vi "Sequence Editor.vi"() -> ()   [LabVIEW 2013, in "Simple Sequence Tools - Editor.lvlib"]
uses:
  Simple Sequence Editor Tool Support.llb/Simple Sequence Tools - Editor.lvlib
  Simple Sequence Editor Tool Support.llb/Simple Sequence Tools - Shared.lvlib
panel:
  in  "Sequence":i32[](listbox)
  in  "NIVS.Workspace Event":refnum<event-registration>
  in  "Iteration Information Channel":string(combo)
  in  "Iterations":u32=1 min=1
  in  "View":enum8{"Step Properties", "Sequence Properties"}(ring)=enum."Sequence Properties"
  in  "Abort Channel":string(combo)
  in  "Step Information Channel":string(combo)
  out "Graph":waveform(dbl)[](graph)
  out "Path":path
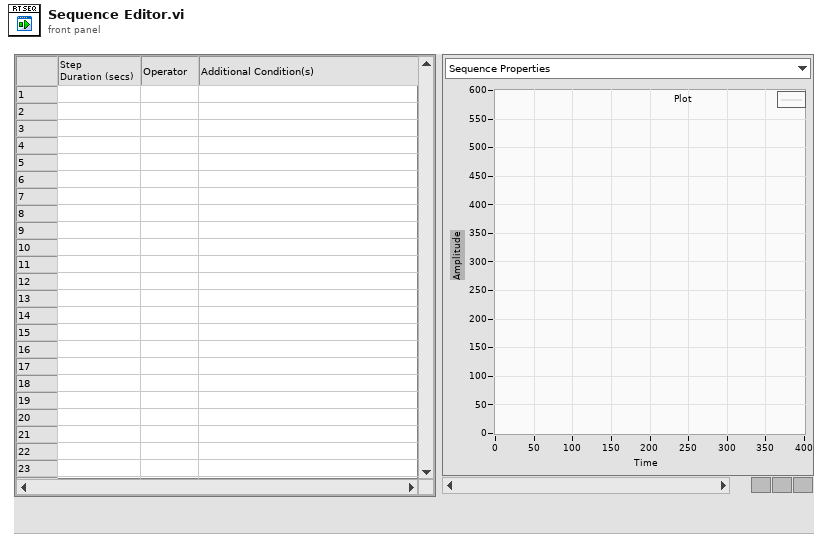
[diagram p1: front panel]
types:
  T1 = cluster{"Aliases.All":cluster{"Name":string, "NodePath":string, "ScaleUnits":string}[], "Aliases.Outputs":cluster{"Name":string, "NodePath":string, "ScaleUnits":string}[], "UI.Sequence#ofColumns":i32, "SysDef.Path":path, "UI.SequenceRef":refnum<vi>, "UI.StepInformationRef":refnum<vi>, "UI.AbortRef":refnum<vi>, "UI.GraphRef":refnum<vi>, "UI.ViewRef":refnum<vi>, "UI.IterationsRef":refnum<vi>, "UI.IterationInformationRef":refnum<vi>, "INI.Settings":cluster{"Build Location":path, "LoggingLocation":path}, "NIVS.Workspace Event":refnum<event-registration>}
  T2 = typedef "LVPoint32TypeDef.ctl" = cluster{"Horizontal":i32, "Vertical":i32}
  T3 = cluster{"Build Location":path, "LoggingLocation":path}
  T4 = cluster{"Name":string, "NodePath":string, "ScaleUnits":string}[]
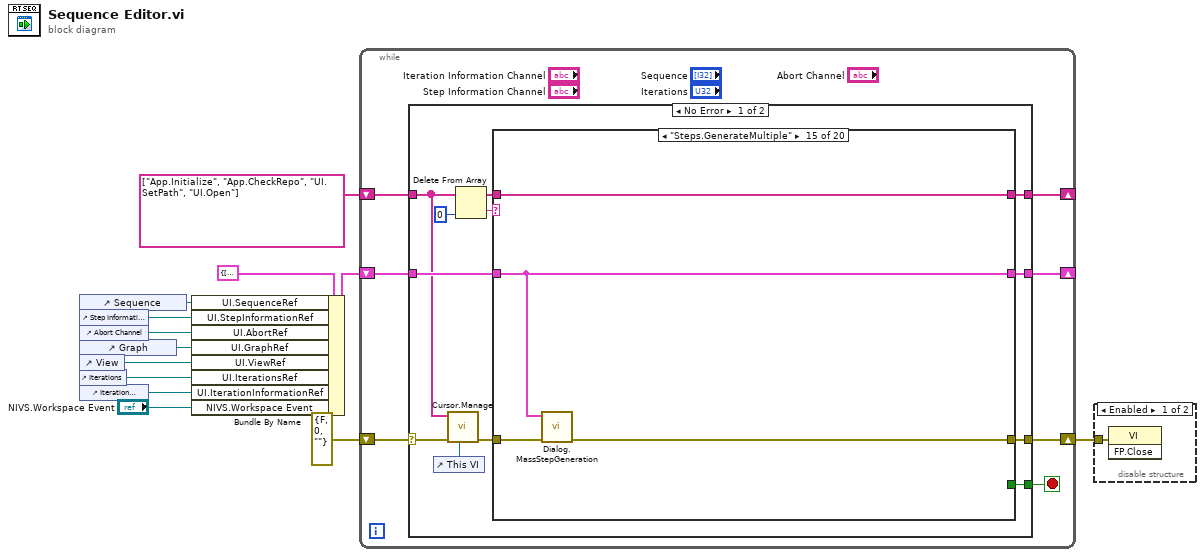
[diagram p0: block diagram]
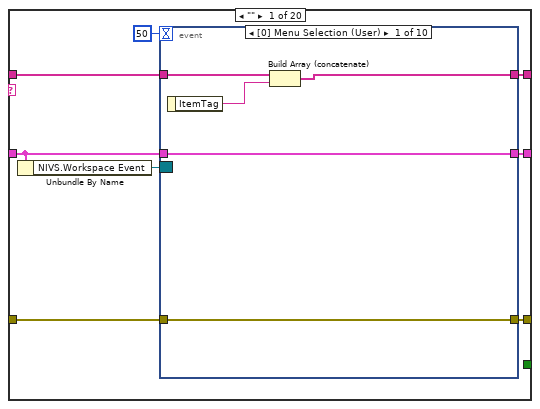
[diagram p3: hidden frame]
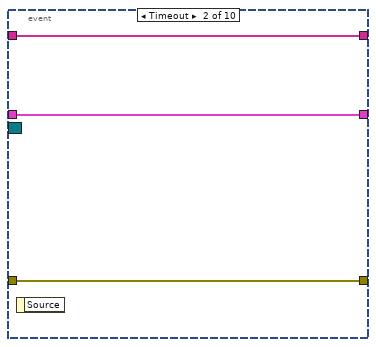
[diagram p4: hidden frame]
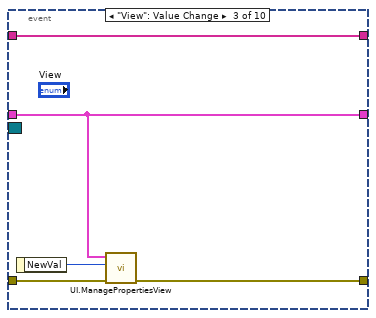
[diagram p5: hidden frame]
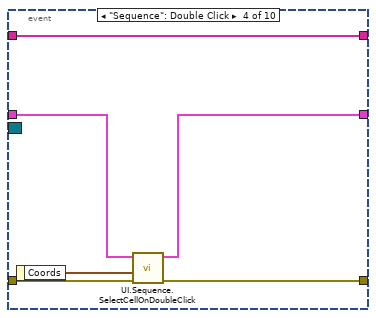
[diagram p6: hidden frame]
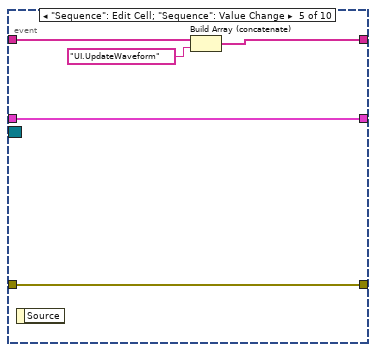
[diagram p7: hidden frame]
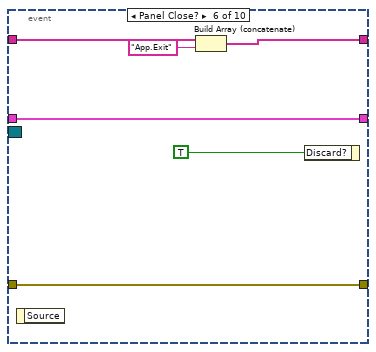
[diagram p8: hidden frame]
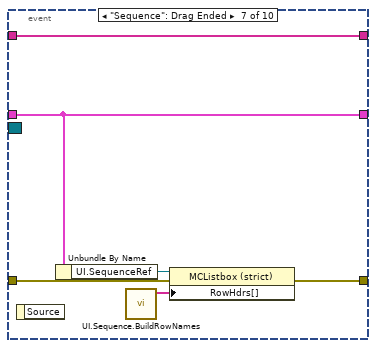
[diagram p9: hidden frame]
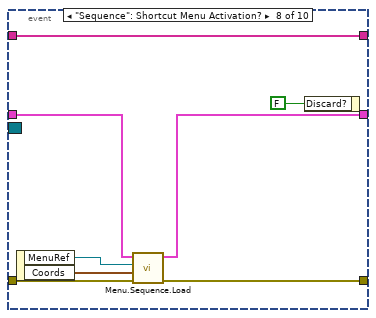
[diagram p10: hidden frame]
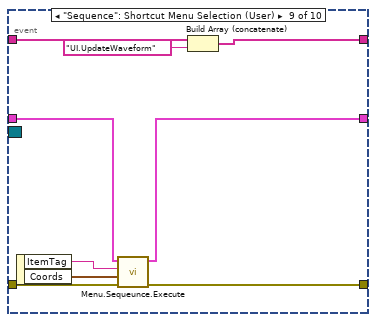
[diagram p11: hidden frame]
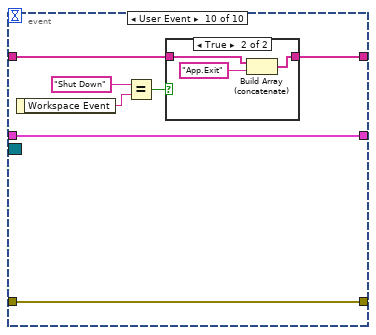
[diagram p12: hidden frame]
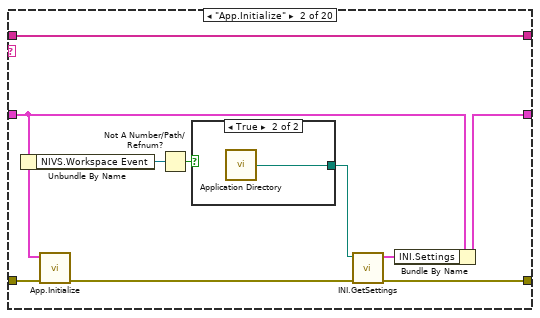
[diagram p14: hidden frame]
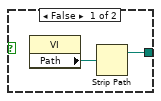
[diagram p15: hidden frame]
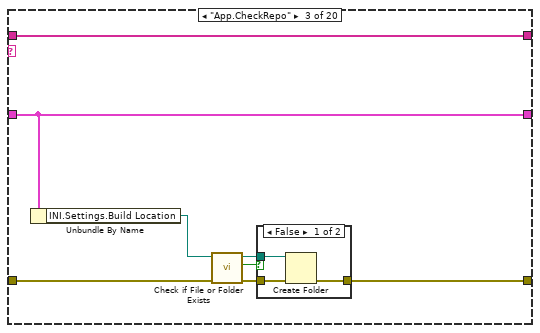
[diagram p16: hidden frame]
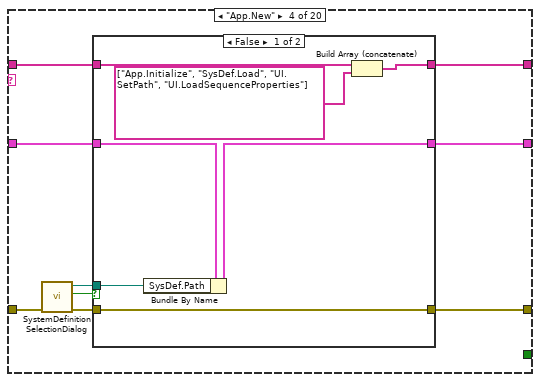
[diagram p18: hidden frame]
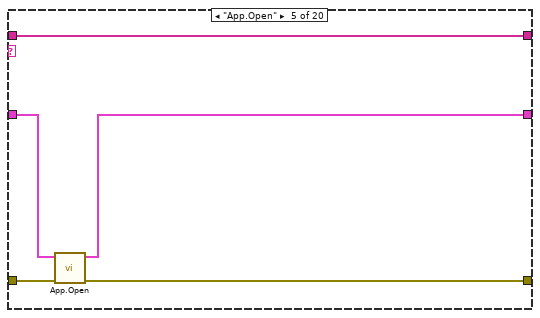
[diagram p20: hidden frame]
diagram:
  n1 = control-ref of="Sequence"() -> (w9:refnum<vi>)
  n2 = control-ref of="Step Information Channel"() -> (w8:refnum<vi>)
  n3 = control-ref of="Abort Channel"() -> (w7:refnum<vi>)
  n4 = control-ref of="Graph"() -> (w6:refnum<vi>)
  n5 = control-ref of="View"() -> (w5:refnum<vi>)
  n6 = control-ref of="Iterations"() -> (w4:refnum<vi>)
  n7 = control-ref of="Iteration Information Channel"() -> (w3:refnum<vi>)
  n8 = Bundle By Name(cluster=T1 {"Aliases.All"=[], "Aliases.Outputs"=[], "UI.Sequence#ofColumns"=0, "SysDef.Path"=path "", "UI.SequenceRef"=refnum, "UI.StepInformationRef"=refnum, "UI.AbortRef"=refnum, "UI.GraphRef"=refnum, "UI.ViewRef"=refnum, "UI.IterationsRef"=refnum, "UI.IterationInformationRef"=refnum, "INI.Settings"={"Build Location"=path "", "LoggingLocation"=path ""}, "NIVS.Workspace Event"=refnum}, "UI.SequenceRef"=w9, "UI.StepInformationRef"=w8, "UI.AbortRef"=w7, "UI.GraphRef"=w6, "UI.ViewRef"=w5, "UI.IterationsRef"=w4, "UI.IterationInformationRef"=w3, "NIVS.Workspace Event"="NIVS.Workspace Event") -> (w10:T1)
  n9 = while {
    shift-right: [w19] -> _
    shift-left: string[] ["App.Initialize", "App.CheckRepo", "UI.SetPath", "UI.Open"] -> [w20]
    shift-right: [w17] -> _
    shift-left: w10 -> [w18]
    shift-right: [w15] -> w2
    shift-left: errorcluster {"status"=FALSE, "code"=0, "source"=""} ("error constant") -> [w16]
    stop <- w14 stop-if-true
    n10 = case shown="No Error" w16 {
      selector: w16 -> [w24 w245]
      tunnel: w20 -> [w25 w248]
      tunnel: [w31 w248] -> w19
      tunnel: w18 -> [w29 w247]
      tunnel: [w28 w247] -> w17
      tunnel: [w27 w244] -> w15
      tunnel: [w26 _] -> w14
      frame No Error {
        n11 = control-ref of="This VI"() -> (w21:refnum<vi>)
        n12 = call "Cursor.Manage.vi"("VI reference (current VI)"=w21, "error in (no error)"=w24, "Cmd list"=w25) -> ("error out"=w23:errorcluster)  [unwired: 8 in]
        n13 = Delete From Array(array=w25, index=0) -> (deleted portion=w32:string, array with subset deleted=w30:string[])  [unwired: 1 in]
        n14 = case shown="\"Steps.GenerateMultiple\"" w32 {
          tunnel: [w38 w114 w125 w130 w153 w157 w161 w168 w179 w183 w184 w210 w214 w218 w223 w227 w233 w237 w240 w243] -> w31
          tunnel: w30 -> [w37 w114 w125 w131 w153 w157 w161 w168 w179 w183 w185 w210 w214 w219 w223 w227 w233 w237 w240 w243]
          tunnel: w29 -> [w34 w105 w124 w134 w150 w155 w160 w165 w178 w180 w188 w207 w213 w215 w220 w225 w229 w236 w239 w242]
          tunnel: [w40 w109 w124 w132 w149 w155 w160 w165 w178 w180 w186 w206 w213 w215 w220 w225 w230 w236 w239 w242] -> w28
          tunnel: [w35 w111 w119 w135 w151 w156 w159 w166 w176 w182 w189 w208 w211 w216 w221 w226 w231 w234 w238 w241] -> w27
          tunnel: w23 -> [w36 w113 w122 w137 w152 w154 w159 w167 w177 w181 w191 w203 w212 w216 w222 w226 w228 w235 w238 w241]
          tunnel: [_ _ _ _ _ _ TRUE _ _ _ _ _ _ _ _ _ _ _ _ _] -> w26
          frame "" {
            n15 = Unbundle By Name(w34) -> ("NIVS.Workspace Event"=w33:refnum<event-registration>)
            n16 = event shown="[0] Menu Selection (User)" {
              selector: w33 -> [_ _ _ _ _ _ _ _ _ _]
              dyn-events: _ -> [_ _ _ _ _ _ _ _ _ _]
              timeout: 50 -> [_ _ _ _ _ _ _ _ _ _]
              tunnel: [w42 w48 w53 w59 w61 w66 w76 w84 w86 w94] -> w38
              tunnel: w37 -> [w44 w48 w53 w59 w64 w70 w76 w84 w93 w95]
              tunnel: [w45 w47 w52 w54 w63 w69 w72 w80 w87 w100] -> w40
              tunnel: w34 -> [w45 w47 w52 w55 w63 w69 w72 w79 w88 w100]
              tunnel: [w43 w46 w49 w56 w62 w68 w73 w81 w89 w99] -> w35
              tunnel: w36 -> [w43 w46 w51 w57 w62 w68 w74 w82 w90 w99]
              event Menu Selection (User) {
                n17 = event-data() -> ("ItemTag"=w41:string)  [unwired: 1 in]
                n18 = Build Array (concatenate)(w44, w41) -> (w42:string[])
              }
              event Timeout {
                n19 = event-data() -> ()  [unwired: 1 in, 1 out]
              }
              event "View": Value Change {
                n20 = event-data() -> ("NewVal"=w50:enum8{"Step Properties", "Sequence Properties"})  [unwired: 1 in]
                n21 = call "UI.ManagePropertiesView.vi"("error in (no error)"=w51, "NewVal"=w50, "State Variables"=w52) -> ("error out"=w49:errorcluster)  [unwired: 8 in]
              }
              event "Sequence": Double Click {
                n22 = event-data() -> ("Coords"=w58:T2)  [unwired: 1 in]
                n23 = call "UI.Sequence.SelectCellOnDoubleClick.vi"("error in (no error)"=w57, "Coords"=w58, "State Variables"=w55) -> ("error out"=w56:errorcluster, "State Variables out"=w54:T1)  [unwired: 7 in]
              }
              event "Sequence": Edit Cell; "Sequence": Value Change {
                n24 = event-data() -> ()  [unwired: 1 in, 1 out]
                n25 = Build Array (concatenate)(w64, "UI.UpdateWaveform" ("message")) -> (w61:string[])
              }
              event Panel Close? {
                n26 = event-data() -> ()  [unwired: 1 in, 1 out]
                n27 = Build Array (concatenate)(w70, "App.Exit") -> (w66:string[])
                n28 = event-data("Discard?"=TRUE) -> ()  [unwired: 1 in, 1 out]
              }
              event "Sequence": Drag Ended {
                n29 = event-data() -> ()  [unwired: 1 in, 1 out]
                n30 = Unbundle By Name(w72) -> ("UI.SequenceRef"=w71:refnum<vi>)
                n31 = call "UI.Sequence.BuildRowNames.vi"() -> ("Row Headings"=w75:string[])  [unwired: 11 in]
                n32 = property class="MCListbox (strict)"(reference=w71, error in=w74, "RowHdrs[]"=w75) -> (error out=w73:errorcluster)  [unwired: 1 out]
              }
              event "Sequence": Shortcut Menu Activation? {
                n33 = event-data() -> ("MenuRef"=w77:refnum<k9>, "Coords"=w78:T2)  [unwired: 1 in]
                n34 = call "Menu.Sequence.Load.vi"("error in (no error)"=w82, "Coords"=w78, "MenuRef"=w77, "State Variables"=w79) -> ("error out"=w81:errorcluster, "State Variables out"=w80:T1)  [unwired: 6 in]
                n35 = event-data("Discard?"=FALSE) -> ()  [unwired: 1 in, 1 out]
              }
              event "Sequence": Shortcut Menu Selection (User) {
                n36 = event-data() -> ("ItemTag"=w92:string, "Coords"=w91:T2)  [unwired: 1 in]
                n37 = call "Menu.Sequeunce.Execute.vi"("error in (no error)"=w90, "Coords"=w91, "ItemPath"=w92, "State Variables"=w88) -> ("error out"=w89:errorcluster, "State Variables out"=w87:T1)  [unwired: 6 in]
                n38 = Build Array (concatenate)(w93, "UI.UpdateWaveform" ("message")) -> (w86:string[])
              }
              event User Event {
                n39 = event-data() -> ("Workspace Event"=w97:string)  [unwired: 1 in]
                n40 = Equal?(x="Shut Down" ("y"), y=w97) -> (x = y?=w96:bool)
                n41 = case shown="True" w96 {
                  tunnel: w95 -> [w101 w103]
                  tunnel: [w101 w102] -> w94
                  frame False {
                  }
                  frame True {
                    n42 = Build Array (concatenate)(w103, "App.Exit") -> (w102:string[])
                  }
                }
              }
            }
          }
          frame "App.Initialize" {
            n43 = Unbundle By Name(w105) -> ("NIVS.Workspace Event"=w108:refnum<event-registration>)
            n44 = call "App.Initialize.vi"("error in (no error)"=w113, "Start Variables"=w105) -> ("error out"=w112:errorcluster)  [unwired: 9 in]
            n45 = Not A Number/Path/Refnum?(number/path/refnum=w108) -> (NaN/Path/Refnum?=w107:bool)
            n46 = case shown="True" w107 {
              tunnel: [w115 w117] -> w106
              frame False {
                n47 = property class="VI"() -> ("Path"=w116:path)  [unwired: 2 in, 2 out]
                n48 = Strip Path(path=w116) -> (stripped path=w115:path)  [unwired: 1 out]
              }
              frame True {
                n49 = call "Application Directory.vi"() -> ("Application Directory"=w117:path)
              }
            }
            n50 = call "INI.GetSettings.vi"("error in (no error)"=w112, "INI Folder Location"=w106) -> ("error out"=w111:errorcluster, "INI.Settings"=w110:T3)  [unwired: 8 in]
            n51 = Bundle By Name(cluster=w105, "INI.Settings"=w110) -> (w109:T1)
          }
          frame "App.CheckRepo" {
            n52 = Unbundle By Name(w124) -> ("INI.Settings.Build Location"=w123:path)
            n53 = call "Check if File or Folder Exists.vi"("error in (no error)"=w122, "path"=w123) -> ("error out"=w120:errorcluster, "file or folder exists?"=w118:bool, "dup path"=w121:path)  [unwired: 7 in]
            n54 = case shown="False" w118 {
              tunnel: w121 -> [w128 _]
              tunnel: w120 -> [w127 w129]
              tunnel: [w126 w129] -> w119
              frame False {
                n55 = Create Folder(path (use dialog)=w128, error in=w127) -> (error out=w126:errorcluster)  [unwired: 1 in, 2 out]
              }
              frame True {
              }
            }
          }
          frame "App.New" {
            n56 = call "SystemDefinitionSelectionDialog.vi"("error in (no error)"=w137) -> ("error out"=w138:errorcluster, "cancelled"=w136:bool, "selected path"=w133:path)  [unwired: 8 in]
            n57 = case shown="False" w136 {
              tunnel: w138 -> [w145 w147]
              tunnel: [w145 w147] -> w135
              tunnel: w134 -> [w144 w148]
              tunnel: [w143 w148] -> w132
              tunnel: w133 -> [w142 _]
              tunnel: [w141 w146] -> w130
              tunnel: w131 -> [w139 w146]
              frame False {
                n58 = Bundle By Name(cluster=w144, "SysDef.Path"=w142) -> (w143:T1)
                n59 = Build Array (concatenate)(w139, string[] ["App.Initialize", "SysDef.Load", "UI.SetPath", "UI.LoadSequenceProperties"]) -> (w141:string[])
              }
              frame True {
              }
            }
          }
          frame "App.Open" {
            n60 = call "App.Open.vi"("error in (no error)"=w152, "State Variables"=w150) -> ("error out"=w151:errorcluster, "State Variables out"=w149:T1)  [unwired: 8 in]
          }
          frame "App.Save" {
            n61 = call "App.Save.vi"("error in (no error)"=w154, "State Variables"=w155) -> ("error out"=w156:errorcluster)  [unwired: 9 in]
          }
          frame "App.Exit" {
          }
          frame "Sequence.Validate" {
            n62 = call "Sequence.Compile.vi"("error in (no error)"=w167, "State Variables"=w165) -> ("error out"=w166:errorcluster, "Warnings"=w162:string[])  [unwired: 7 in, 1 out]
            n63 = Empty Array?(array=w162) -> (empty?=w164:bool)
            n64 = case shown="True" w164 {
              tunnel: [w172 "Configuration Valid"] -> w163
              tunnel: w162 -> [w173 _]
              frame False {
                n65 = Array To Spreadsheet String(delimiter (Tab)="\r\n", array=w173, 3:"%s" ("format string")) -> (spreadsheet string=w171:string)
                n66 = Concatenate Strings("Configuration Contains Errors:\n\n", w171) -> (w172:string)
              }
              frame True {
              }
            }
            n67 = One Button Dialog(message=w163) -> ()  [unwired: 1 in, 1 out]
          }
          frame "Sequence.Preview" {
            n68 = call "Sequence.Preview.vi"("error in (no error)"=w177, "State Variables"=w178) -> ("error out"=w176:errorcluster)  [unwired: 9 in]
          }
          frame "Sequence.Build" {
            n69 = call "Sequence.Build.vi"("error in (no error)"=w181, "State Variables"=w180) -> ("error out"=w182:errorcluster)  [unwired: 9 in]
          }
          frame "SysDef.New" {
            n70 = call "SystemDefinitionSelectionDialog.vi"("error in (no error)"=w191) -> ("error out"=w192:errorcluster, "cancelled"=w190:bool, "selected path"=w187:path)  [unwired: 8 in]
            n71 = case shown="False" w190 {
              tunnel: w192 -> [w199 w201]
              tunnel: [w199 w201] -> w189
              tunnel: w188 -> [w198 w202]
              tunnel: [w197 w202] -> w186
              tunnel: w187 -> [w196 _]
              tunnel: [w195 w200] -> w184
              tunnel: w185 -> [w193 w200]
              frame False {
                n72 = Bundle By Name(cluster=w198, "SysDef.Path"=w196) -> (w197:T1)
                n73 = Build Array (concatenate)(w193, string[] ["SysDef.Load", "UI.SetPath", "UI.LoadSequenceProperties"]) -> (w195:string[])
              }
              frame True {
              }
            }
          }
          frame "SysDef.Load" {
            n74 = Unbundle By Name(w207) -> ("SysDef.Path"=w209:path)
            n75 = call "LoadSystemDefinition.vi"("error in (no error)"=w203, "SysDef.Path"=w209) -> ("error out"=w208:errorcluster, "Aliases.Outputs"=w204:T4, "Aliases.All"=w205:T4)  [unwired: 7 in]
            n76 = Bundle By Name(cluster=w207, "Aliases.All"=w205, "Aliases.Outputs"=w204) -> (w206:T1)
          }
          frame "SysDef.Edit" {
            n77 = call "SysDef.Edit.vi"("error in (no error)"=w212, "State Variables"=w213) -> ("error out"=w211:errorcluster)  [unwired: 9 in]
          }
          frame "SysDef.Refresh" {
            n78 = Build Array (concatenate)(w219, string[] ["SysDef.Load", "UI.SetPath", "UI.LoadSequenceProperties"]) -> (w218:string[])
          }
          frame "Steps.GenerateMultiple" {
            n79 = call "Dialog.MassStepGeneration.vi"("error in (no error)"=w222, "State Variables"=w220) -> ("error out"=w221:errorcluster)  [unwired: 9 in]
          }
          frame "UI.SetPath" {
            n80 = Unbundle By Name(w225) -> ("SysDef.Path"=→"Path":path)
          }
          frame "UI.UpdateWaveform" {
            n81 = call "UI.UpdateWaveform.vi"("error in (no error)"=w228, "State Variables"=w229) -> ("error out"=w231:errorcluster, "Wavefrom"=→"Graph":waveform(dbl)[], "State Variables out"=w230:T1)  [unwired: 7 in]
          }
          frame "UI.LoadSequenceProperties" {
            n82 = call "UI.LoadComboBoxes.vi"("error in (no error)"=w235, "State Variables"=w236) -> ("error out"=w234:errorcluster)  [unwired: 9 in]
          }
          frame "UI.Open" {
            n83 = invoke class="VI" method="FP.Open"() -> ()  [unwired: 5 in, 5 out]
          }
          frame Default {
          }
        }
      }
      frame Error {
        n84 = call "Simple Error Handler.vi"("error in (no error)"=w245) -> ("error out"=w246:errorcluster)  [unwired: 4 in, 4 out]
        n85 = call "Clear Errors.vi"("error in (no error)"=w246) -> ("error out"=w244:errorcluster)  [unwired: 6 in]
      }
    }
  }
  n86 = disable-structure shown="Enabled" {
    disable-tunnel: w2 -> [w249 _]
    frame Enabled {
      n87 = invoke class="VI" method="FP.Close"(error in=w249) -> ()  [unwired: 2 in, 3 out]
    }
    frame Disabled {
    }
  }
